vi "main_save_camera_images.vi"(8 "error in (no error)":errorcluster, 9 "Median Filtered Image":T2, 10 "Session In":T1, 11 "Queue in":refnum<queue>) -> (0 "error out":errorcluster, 3 "Decoded Camera Frmes":i32[](array[numeric]))   [LabVIEW 2019]
uses:
  <vilib>/vision/Image Controls.llb/IMAQ Image.ctl
  <vilib>/userDefined/High Color/IMAQdx.ctl
  <vilib>/vision/driver/IMAQdx.llb/IMAQdx Buffer Number Mode.ctl
  TimestampsFunctionalGlobalOperations.ctl
  ParametersGlobal.vi
  DebugGlobal.vi
  <vilib>/vision/driver/NI_Vision_Acquisition_Software.lvlib
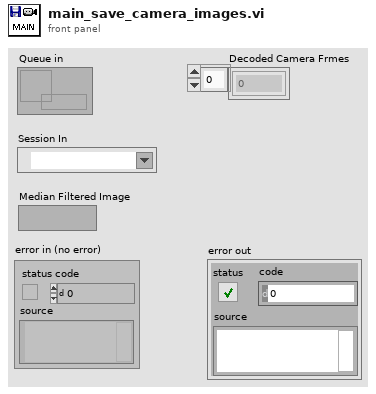
[diagram p1: front panel]
types:
  T1 = typedef "IMAQdx.ctl" = refnum<k21>
  T2 = typedef "IMAQ Image.ctl" = refnum<image>
  T3 = typedef "Image Type" = u32
  T4 = typedef "NI_Vision_Acquisition_Software.lvlib/IMAQdx Buffer Number Mode.ctl" = enum32{"Next", "Last", "Buffer Number", "Every", "Last New"}
  T5 = typedef "TimestampsFunctionalGlobalOperations.ctl" = enum16{"Initialize", "Dump", "UpdateTime", "ReadTime"}
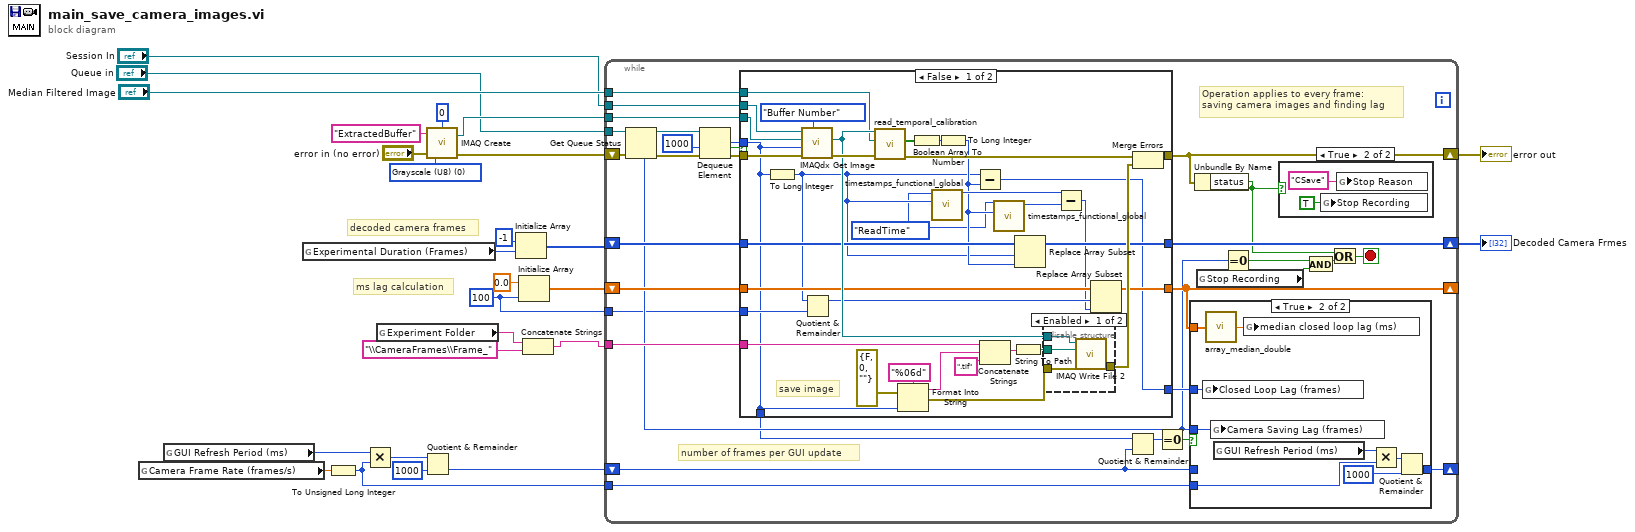
[diagram p0: block diagram]
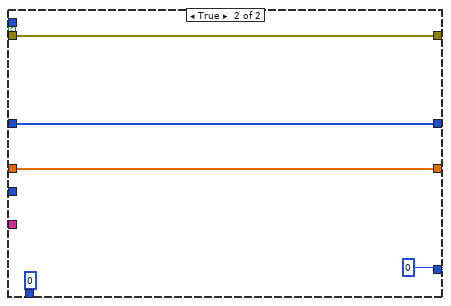
[diagram p5: hidden frame]
diagram:
  w16 = 100 ("dimension size")
  w15 = T3 0 items=["Grayscale (U8)", "Grayscale (I16)", "Grayscale (SGL)", "Complex (CSG)", "RGB (U32)", "HSL (U32)", "RGB (U64)"] ("Image Type")
  # "ms lag calculation"
  # "decoded camera frames"
  n1 = global read "ParametersGlobal.vi" "Camera Frame Rate (frames/s)"() -> (w21:sgl)
  n2 = global read "DebugGlobal.vi" "GUI Refresh Period (ms)"() -> (w23:u32)
  n3 = global read "ParametersGlobal.vi" "Experimental Duration (Frames)"() -> (w8:i32)
  n4 = To Unsigned Long Integer(number=w21) -> (unsigned 32bit integer=w2:u32)
  n5 = Multiply(x=w23, y=w2) -> (x*y=w22:u32)
  n6 = global read "ParametersGlobal.vi" "Experiment Folder"() -> (w9:string)
  n7 = Quotient & Remainder(x=w22, y=u32 1000) -> (floor(x/y)=w25:u32)  [unwired: 1 out]
  n8 = call "IMAQ Create"("Border Size"=0, "Image Name"="ExtractedBuffer", "Image Type"=w15, "error in (no error)"="error in (no error)") -> ("New Image"=w20:T2, "error out"=w26:errorcluster)  [unwired: 1 in]
  n9 = Initialize Array(-1, w8) -> (w18:i32[])
  n10 = Initialize Array(0.0 ("x-y"), w16) -> (w17:dbl[])
  n11 = Concatenate Strings(w9, "\\CameraFrames\\Frame_" ("string")) -> (w19:string)
  n12 = while {
    shift-right: [w47] -> w3
    shift-left: w26 -> [w52]
    tunnel: "Session In" -> [w55]
    tunnel: "Queue in" -> [w54]
    tunnel: w20 -> [w53]
    tunnel: w19 -> [w45]
    tunnel: "Median Filtered Image" -> [w42]
    shift-right: [w40] -> w7
    shift-left: w18 -> [w41]
    shift-right: [w38] -> _
    shift-left: w17 -> [w39]
    tunnel: w16 -> [w30]
    shift-right: [w36] -> _
    shift-left: w25 -> [w34]
    tunnel: w2 -> [w27]
    stop <- w48 stop-if-true
    # "number of frames per GUI update"
    # "Operation applies to every frame: \nsaving camera images and finding lag"
    n13 = Get Queue Status(queue=w54, error in (no error)=w52) -> (queue out=w57:refnum<queue>, error out=w51:errorcluster, # elements in queue=w35:i32)  [unwired: 1 in, 5 out]
    n14 = Dequeue Element(queue=w57, timeout in ms (-1)=1000, error in (no error)=w51) -> (element=w46:u32, timed out?=w43:bool, error out=w50:errorcluster)  [unwired: 1 out]
    n15 = case shown="False" w43 {
      tunnel: w55 -> [w102 _]
      tunnel: w53 -> [w101 _]
      tunnel: w50 -> [w100 w113]
      tunnel: [w89 w113] -> w47
      tunnel: w46 -> [w72 _]
      tunnel: w45 -> [w93 _]
      tunnel: w42 -> [w70 _]
      tunnel: w41 -> [w82 w112]
      tunnel: [w80 w112] -> w40
      tunnel: w39 -> [w79 w111]
      tunnel: w30 -> [w78 _]
      tunnel: [w75 w111] -> w38
      tunnel: [w73 0] -> w37
      tunnel: [w72 u32 0] -> w31
      frame False {
        w71 = TimestampsFunctionalGlobalOperations."ReadTime" ("Operation")
        # "save image"
        n16 = To Long Integer(number=w72) -> (32bit integer=w77:i32)
        n17 = call <vilib>:"IMAQdx Get Image.vi"("Buffer Number Mode (Next)"=IMAQdx_Buffer_Number_Mode."Buffer Number", "error in"=w100, "Buffer Number In"=w72, "Image In"=w101, "Session In"=w102) -> ("error out"=w91:errorcluster, "Image Out"=w90:T2)  [unwired: 3 in, 2 out]
        n18 = Quotient & Remainder(x=w77, y=w78) -> (x-y*floor(x/y)=w76:i32)  [unwired: 1 out]
        n19 = call "read_temporal_calibration.vi"("error in (no error)"=w91, "Median Filtered Image"=w70, "Aquired Image"=w90) -> ("error out"=w88:errorcluster, "Time Bits Decoded"=w92:bool[])  [unwired: 6 in, 1 out]
        n20 = Format Into String(format string="%06d" ("string"), error in=errorcluster {"status"=FALSE, "code"=0, "source"=""}, w72) -> (resulting string=w94:string, error out=w95:errorcluster)  [unwired: 1 in]
        n21 = Boolean Array To Number(Boolean array=w92) -> (number=w83:u64)
        n22 = call "timestamps_functional_global.vi"("Buffer Number"=w77, "Operation"=w71) -> ("Timestamp Out"=w85:u32)  [unwired: 3 in, 2 out]
        n23 = To Long Integer(number=w83) -> (32bit integer=w81:i32)
        n24 = Subtract(x=w77, y=w81) -> (x-y=w73:i32)
        n25 = Concatenate Strings(w93, w94, ".tif" ("string")) -> (w98:string)
        n26 = call "timestamps_functional_global.vi"("Buffer Number"=w81, "Operation"=w71) -> ("Timestamp Out"=w84:u32)  [unwired: 3 in, 2 out]
        n27 = String To Path(string=w98) -> (path=w97:path)
        n28 = Replace Array Subset(array=w82, new element=w81, index=w77) -> (w80:i32[])
        n29 = disable-structure shown="Enabled" {
          disable-tunnel: w97 -> [w107 _]
          disable-tunnel: [w106 w108] -> w87
          disable-tunnel: w95 -> [w105 w108]
          disable-tunnel: w90 -> [w104 _]
          frame Enabled {
            n30 = call-poly "IMAQ Write File 2"("error in (no error)"=w105, "File Path"=w107, "Image"=w104) -> ("error out"=w106:errorcluster)  [unwired: 7 in, 1 out]
          }
          frame Disabled {
          }
        }
        n31 = Subtract(x=w85, y=w84) -> (x-y=w74:u32)
        n32 = Replace Array Subset(array=w79, new element=w74, index=w76) -> (w75:dbl[])
        n33 = Merge Errors(w88, w87) -> (w89:errorcluster)
      }
      frame True {
      }
    }
    n34 = Quotient & Remainder(x=w31, y=w34) -> (x-y*floor(x/y)=w33:u32)  [unwired: 1 out]
    n35 = Equal To 0?(x=w33) -> (x = 0?=w32:bool)
    n36 = case shown="True" w32 {
      tunnel: w38 -> [_ w65]
      tunnel: w35 -> [_ w62]
      tunnel: w37 -> [_ w63]
      tunnel: [w60 w66] -> w36
      tunnel: w34 -> [w60 _]
      tunnel: w27 -> [_ w61]
      frame False {
      }
      frame True {
        n37 = global write "DebugGlobal.vi" "Closed Loop Lag (frames)"(w63) -> ()
        n38 = call "array_median_double.vi"("Input Array"=w65) -> ("Median"=w64:dbl)
        n39 = global write "DebugGlobal.vi" "Camera Saving Lag (frames)"(w62) -> ()
        n40 = global read "DebugGlobal.vi" "GUI Refresh Period (ms)"() -> (w69:u32)
        n41 = global write "DebugGlobal.vi" "median closed loop lag (ms)"(w64) -> ()
        n42 = Multiply(x=w69, y=w61) -> (x*y=w67:u32)
        n43 = Quotient & Remainder(x=w67, y=u32 1000) -> (floor(x/y)=w66:u32)  [unwired: 1 out]
      }
    }
    n44 = Unbundle By Name(w47) -> ("status"=w29:bool)
    n45 = global read "DebugGlobal.vi" "Stop Recording"() -> (w28:bool)
    n46 = Equal To 0?(x=w35) -> (x = 0?=w56:bool)
    n47 = case shown="True" w29 {
      frame False {
      }
      frame True {
        n48 = global write "DebugGlobal.vi" "Stop Recording"(TRUE ("stop")) -> ()
        n49 = global write "DebugGlobal.vi" "Stop Reason"("CSave" ("Stop Debug")) -> ()
      }
    }
    n50 = And(x=w56, y=w28) -> (x .and. y?=w49:bool)
    n51 = Or(x=w29, y=w49) -> (x .or. y?=w48:bool)
  }
  "Decoded Camera Frmes" <- w7
  "error out" <- w3
